vi "PH_ImageOperator.ProcCases.vi"(0 "i ref in":refnum<vi>, 1 "selector":string, 2 "data":T1, 3 "call cluster":T2={"Object"="", "Selector"="", "CallType"=enum."synchronous", "Async Object"="", "Async Selector"="", "Data Descriptor"="", "Data"=[], "Error #"=0, "Expire"=0}, 5 "error in":errorcluster) -> (14 "i ref out":refnum<vi>, 17 "answer cluster":T2={"Object"="", "Selector"="", "CallType"=enum."synchronous", "Async Object"="", "Async Selector"="", "Data Descriptor"="", "Data"=[], "Error #"=0, "Expire"=0}, 19 "error out":errorcluster)   [LabVIEW 2014, in "PH_ImageOperator.lvlib"]
doc: "This method is called by a process from within the default case in the event loop. The methods of a class that are linked to events will be called from THIS method. Add your code here."
uses:
  PH_ImageOperator.lvlib
  CSCore/CSSystem/CoreDefs/CoreDefs.call_type.ctl
  CSCore/BaseProcess/BaseProcess.descriptor string definition.ctl
  CSCore/CSSystem/CoreDefs/CoreDefs.rawDataType.ctl
  CSCore/CSSystem/CoreLib/CoreLib.byte array 2 short.vi
  CSCore/CSSystem/CoreLib/CoreLib.byte array 2 double.vi
  CSCore/CSSystem/CoreLib/CoreLib.string 2 byte array.vi
  CSCore/CSSystem/CoreLib/CoreLib.byte array 2 int.vi
  CSCore/CSSystem/CoreLib/CoreLib.lvlib
  CSCore/BaseProcess/BaseProcess.lvlib
  CSCore/CAEObj/CAEObj.lvlib
  PH_PSDBWriter/PH_PSDBWriter.lvlib
  PH_Common/PH_Common.lvlib
  PH_Img_BaseClass/PH_Img_BaseClass.lvlib
  PH_Cam_BaseClass/PH_Cam_BaseClass.lvlib
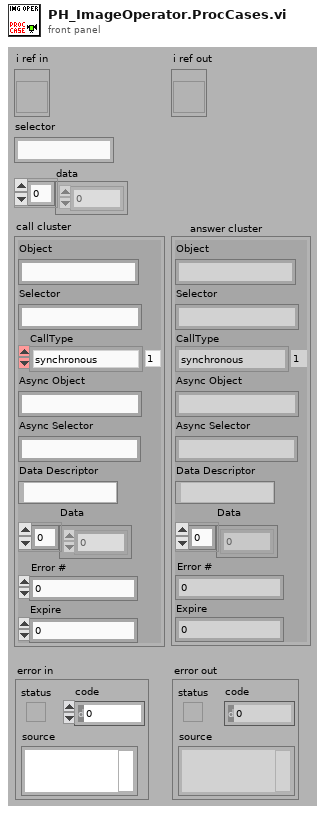
[diagram p1: front panel]
types:
  T1 = typedef "CoreDefs.rawDataType.ctl" = i8[]
  T2 = typedef "CoreDefs.call_type.ctl" = cluster{"Object":string, "Selector":string, "CallType":enum16{"simple", "synchronous", "asynchronous"}, "Async Object":string, "Async Selector":string, "Data Descriptor":T3, "Data":T1, "Error #":i32, "Expire":u32}
  T3 = typedef "BaseProcess.lvlib/BaseProcess.descriptor string definition.ctl" = string
  T4 = typedef "PH_Cam_BaseClass.lvlib/PH_Cam_BaseClass.Settings.ctl" = cluster{"Cam ID":string, "Gain":dbl, "Brightness":dbl, "Shutter":dbl, "Mode":i32}
  T5 = typedef "PH_ImageOperator.lvlib/PH_ImageOperator.i attribute.ctl" = cluster{"GUI Refs":cluster{"Delete":refnum<vi>, "Calibration status":refnum<vi>, "BI subtracted":refnum<vi>, "calc Energy":refnum<vi>, "Energy: expected value":refnum<vi>, "Energy: Tolerance":refnum<vi>, "Energy calculated":refnum<vi>, "Energy":refnum<vi>, "calc Beam Anal":refnum<vi>, "Maj Diam 1/esquare":refnum<vi>, "Min Diam 1/esquare":refnum<vi>, "Azi Angle":refnum<vi>, "Min/Maj Diam esquare":refnum<vi>, "Beam analysed":refnum<vi>, "CoG - x":refnum<vi>, "CoG - y":refnum<vi>, "BA: Method":refnum<vi>, "BA: Steps":refnum<vi>, "BA: Factor":refnum<vi>, "calc Traces":refnum<vi>, "Traces: Fit Gauss":refnum<vi>, "Traces calculated":refnum<vi>, "Maj FWHM":refnum<vi>, "Min FWHM":refnum<vi>, "Major Trace":refnum<vi>, "Minor Trace":refnum<vi>, "Maj Fit Order":refnum<vi>, "Min Fit Order":refnum<vi>, "Position calculated":refnum<vi>, "Position":refnum<vi>, "Type":refnum<vi>, "Center":refnum<vi>, "exp - X":refnum<vi>, "exp - Y":refnum<vi>, "Tolerance":refnum<vi>, "f":refnum<vi>, "M":refnum<vi>, "D":refnum<vi>, "q":refnum<vi>, "Dummy Method":refnum<vi>, "Dummy Type":refnum<vi>, "Global On":refnum<vi>, "Traces: No offset":refnum<vi>, "Maj 99%":refnum<vi>, "Min 99%":refnum<vi>, "GUI FF Image":refnum<vi>, "calc Fill Factor":refnum<vi>, "FF calculated":refnum<vi>, "Fill Factor: Filter?":refnum<vi>, "FF: Damage Threshold":refnum<vi>, "FF: Threshold":refnum<vi>, "FF: max allow. Energy":refnum<vi>, "FF: Fillfactor":refnum<vi>, "Calibration data":refnum<vi>}, "List of GUIs":string[], "Calibration":cluster{"Status":T6, "Calibration data":T7, "Calibration Data File":path}, "Final Image":cluster{"BI Subtraction Failure":bool}, "Energy":cluster{"on":bool, "expected value [mJ]":dbl, "Tolerance [%]":dbl, "State":T6, "Energy [mJ]":dbl, "Unit":string, "calculated @":timestamp}, "Beam Analysis":cluster{"on":bool, "Data":T8, "Method":bool, "Steps":i32, "Factor":i32, "ROI":cluster{"Left":i32, "Top":i32, "Right":i32, "Bottom":i32}, "analysed @":timestamp}, "Trace Analysis":cluster{"on":bool, "Fit on":bool, "Maj FWHM":dbl, "Min FWHM":dbl, "Maj Fit Order":i32, "Min Fit Order":i32, "No Offset":bool, "Maj 99%":dbl, "Min 99%":dbl, "Traces":cluster{"XScaleName":string, "Y Scale Minimum":sgl, "Y Scale Maximum":sgl, "X Scale Minimum":sgl, "X Scale Maximum":sgl, "Traces":cluster{"Index":sgl[], "Trace":dbl[]}[]}[], "analysed @":timestamp}, "Position Analysis":cluster{"on":bool, "exp - X":i32, "exp - Y":i32, "focal length [mm]":dbl, "Magnification":dbl, "Delta":dbl, "Theta":dbl, "Tolerance":dbl, "Type":bool, "analysed @":timestamp}, "Fill Factor":cluster{"on":bool, "Filter on?":bool, "Threshold":dbl, "Damage Threshold [J/cm²]":dbl, "Fillfactor":dbl, "Max. allowed Energy [J]":dbl, "calculated @":timestamp}, "Statistician Service ID":i32, "Images":cluster{"Background":T9, "OP":T9, "GUI":T9, "BA: ROI":T9, "Trace: Turn":T9, "FF: Main":T9, "FF: Help":T9, "PSDB: BG":T9, "PSDB: OP":T9, "PSDB: FF":T9}}
  T6 = typedef "PH_StatusHandler.lvlib/PH_StatusHandler.Status.ctl" = i16
  T7 = typedef "PH_ImageCalibrator.lvlib/PH_ImageCalibrator.Calibration Data.ctl" = cluster{"Date":string, "Time":string, "Cam Settings":cluster{"Cam ID":string, "Gain":dbl, "Brightness":dbl, "Shutter":dbl, "Cam Error":bool, "Mode":i32}, "Background Image":cluster{"Image":dbl[][], "Image Error":bool}, "Linear Calibration":cluster{"Calibration Factor":dbl, "not mm or mrad":bool}, "Energy Calibration":cluster{"Calibration Factor":dbl, "no mJ":bool}}
  T8 = typedef "PH_ImageOperator.lvlib/PH_ImageOperator.Beam Analysis Data.ctl" = cluster{"CoG-x":sgl, "CoG-y":sgl, "Maj Dim":dbl, "Min Dim":dbl, "Ellipticity":dbl, "Azimuth Angle [rad]":dbl, "Azi Angle rel to Maj?":bool}
  T9 = typedef "IMAQ Image.ctl" = refnum<image>
  T10 = typedef "PH_PSDBWriter.lvlib/PH_PSDBWriter.PHELIX-Subsystems.ctl" = i32
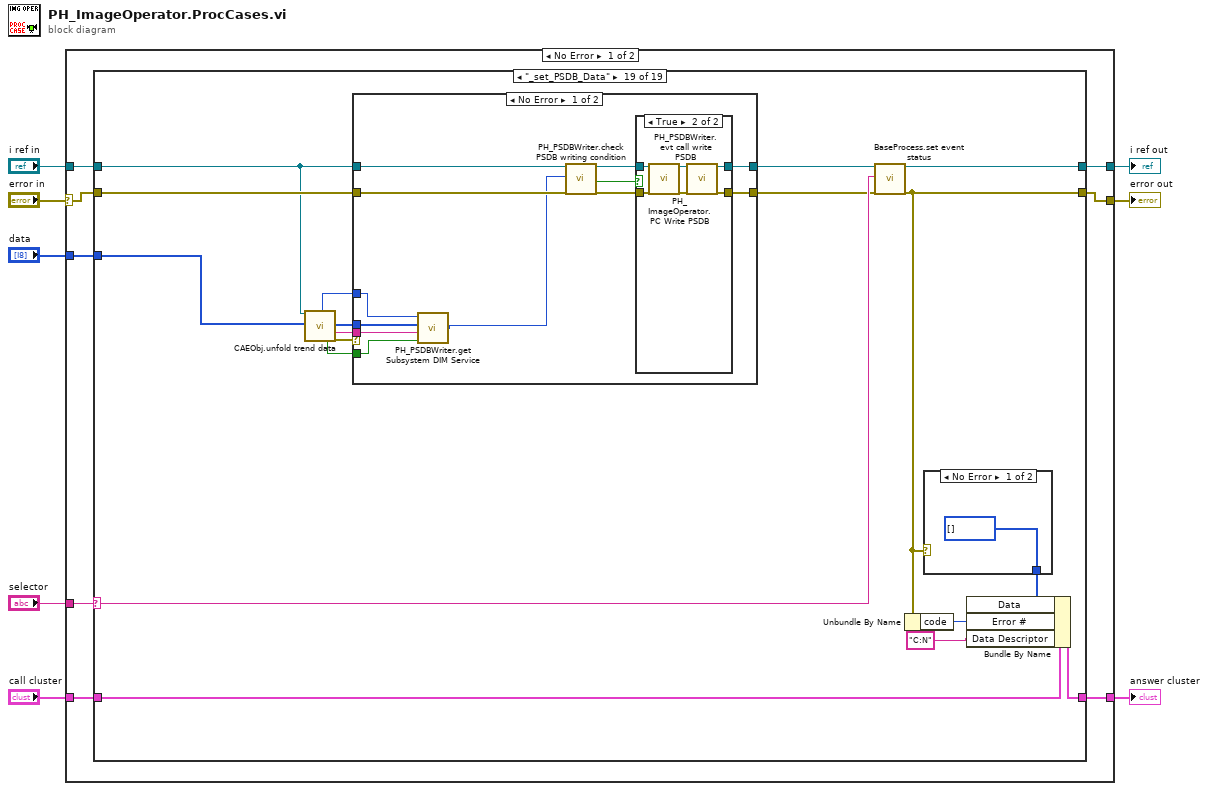
[diagram p0: block diagram]
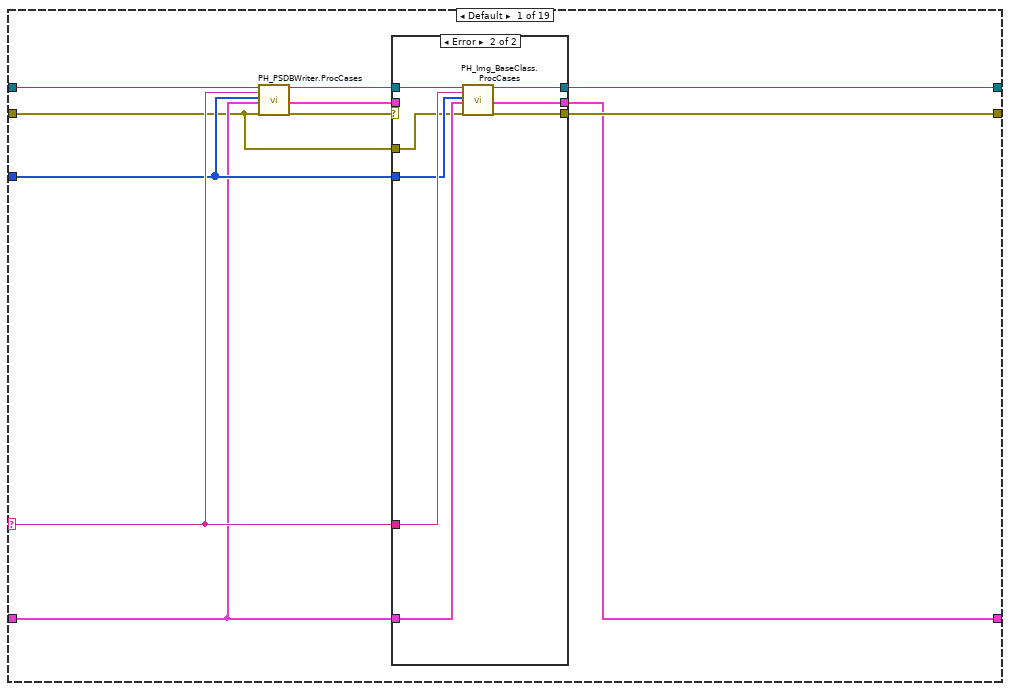
[diagram p2: hidden frame]
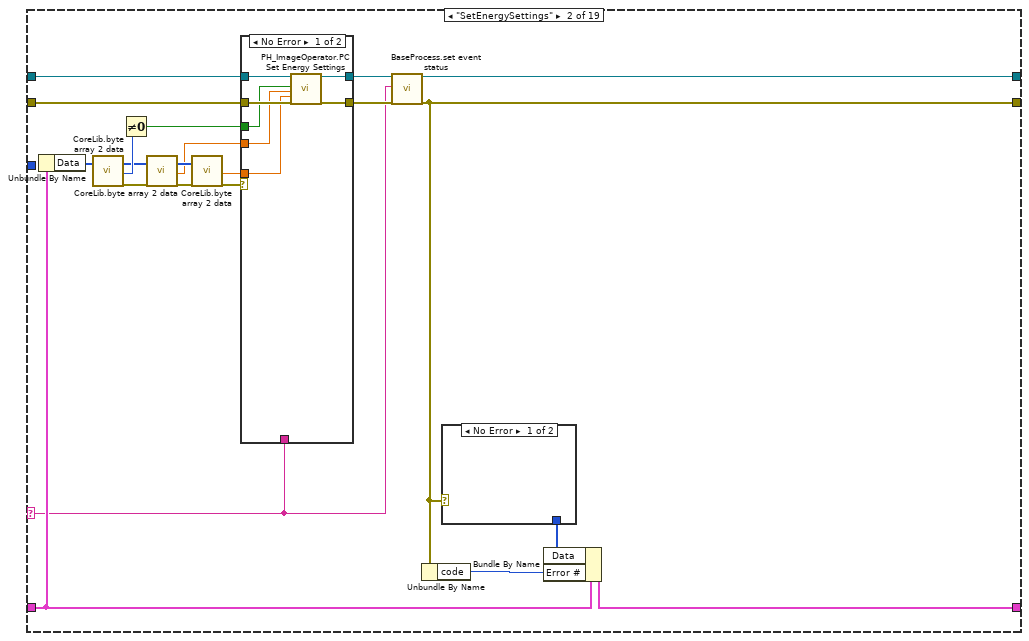
[diagram p4: hidden frame]
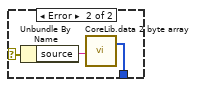
[diagram p5: hidden frame]
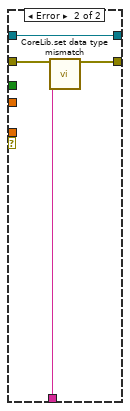
[diagram p6: hidden frame]
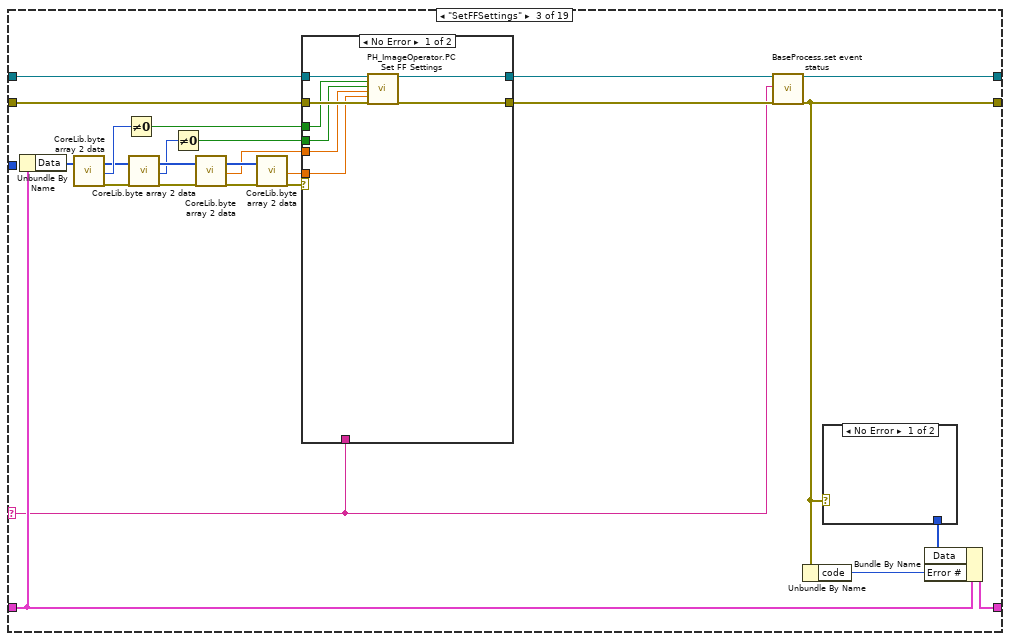
[diagram p7: hidden frame]
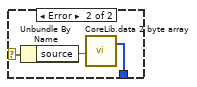
[diagram p8: hidden frame]
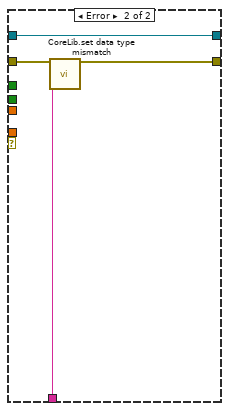
[diagram p9: hidden frame]
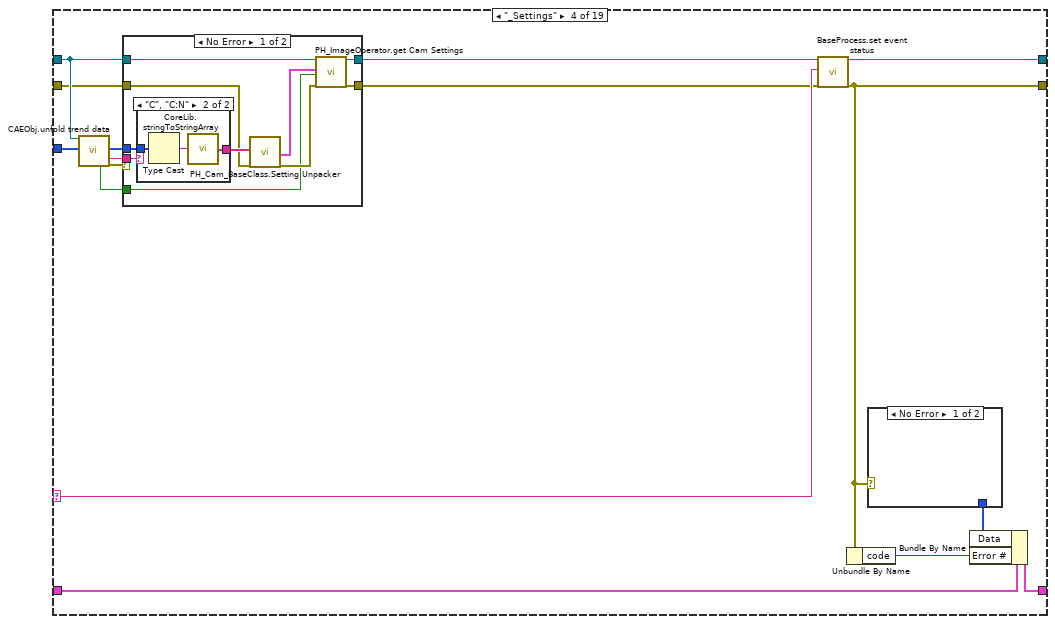
[diagram p10: hidden frame]
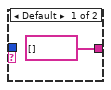
[diagram p11: hidden frame]
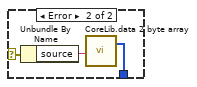
[diagram p13: hidden frame]
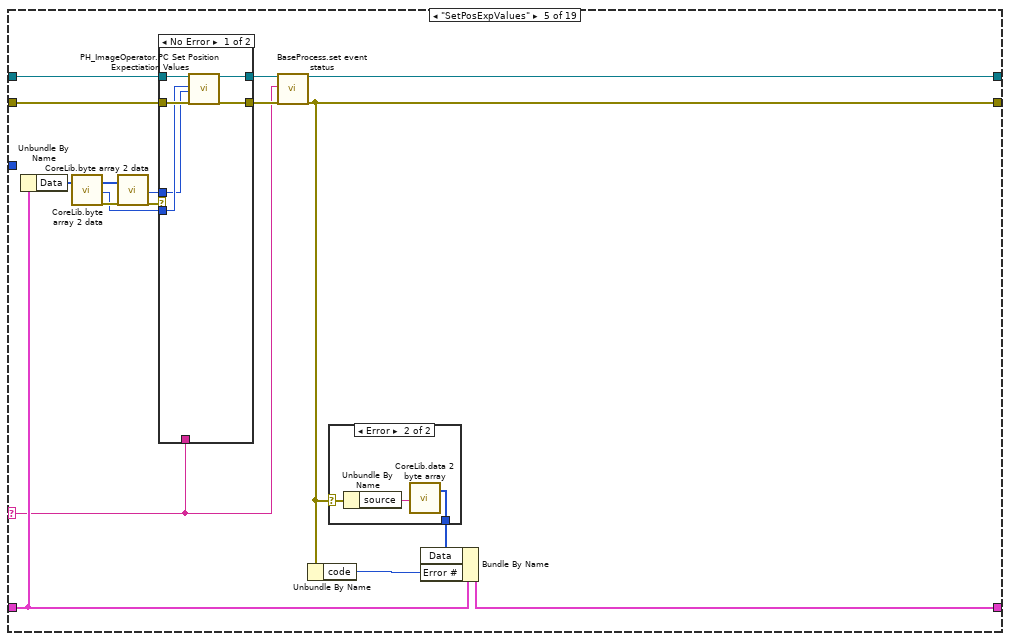
[diagram p14: hidden frame]
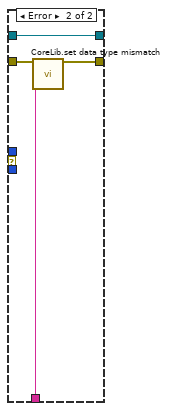
[diagram p16: hidden frame]
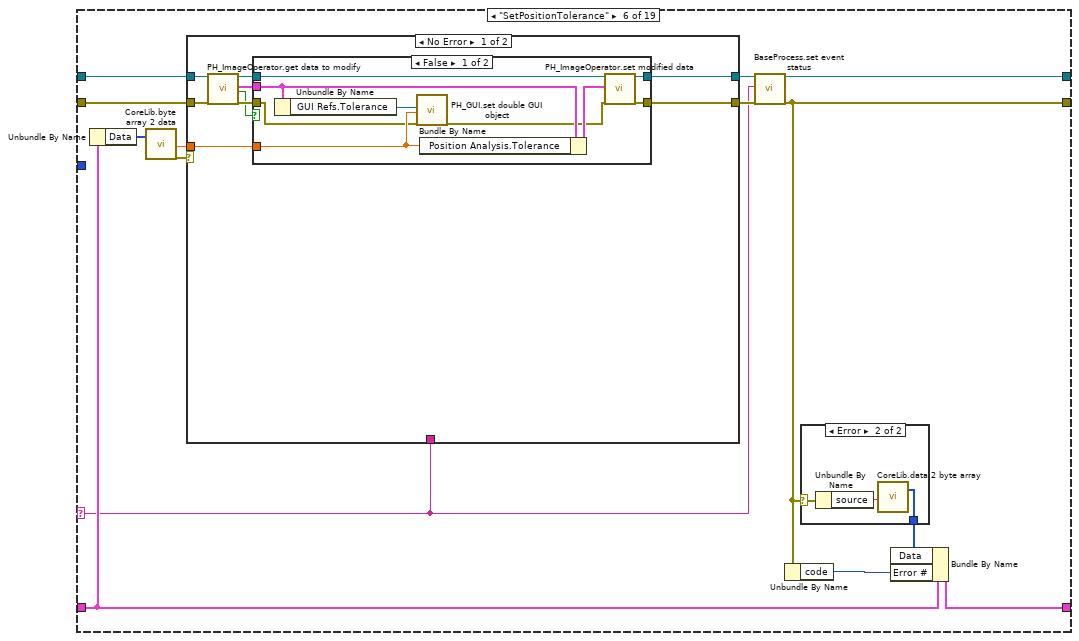
[diagram p17: hidden frame]
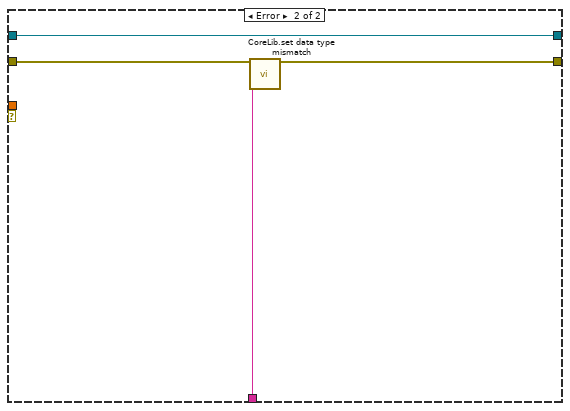
[diagram p20: hidden frame]
diagram:
  n1 = case shown="No Error" "error in" {
    selector: "error in" -> [w9 w619]
    tunnel: "selector" -> [w16 _]
    tunnel: [w15 w618] -> w7
    tunnel: "call cluster" -> [w14 w618]
    tunnel: "i ref in" -> [w13 w620]
    tunnel: [w12 w620] -> w5
    tunnel: [w11 w619] -> w4
    tunnel: "data" -> [w10 _]
    frame No Error {
      n2 = case shown="\"_set_PSDB_Data\"" w16 {
        selector: w16 -> [w22 w51 w90 w125 w157 w184 w225 w266 w314 w343 w370 w397 w424 w464 w485 w512 w539 w566 w586]
        tunnel: w10 -> [w21 _ _ w114 _ _ _ _ _ _ _ _ _ _ _ _ _ _ w574]
        tunnel: w13 -> [w27 w59 w98 w118 w165 w192 w233 w274 w322 w351 w378 w405 w432 w462 w493 w520 w547 w564 w577]
        tunnel: [w24 w50 w89 w124 w156 w183 w224 w265 w313 w342 w369 w396 w423 w463 w484 w511 w538 w565 w587] -> w12
        tunnel: w14 -> [w20 w56 w95 w128 w162 w189 w230 w271 w319 w348 w375 w402 w429 w469 w490 w517 w544 w569 w590]
        tunnel: [w18 w55 w94 w127 w161 w188 w229 w270 w318 w347 w374 w401 w428 w468 w489 w516 w543 w568 w589] -> w15
        tunnel: w9 -> [w17 w58 w97 w116 w164 w191 w232 w273 w321 w350 w377 w404 w431 w460 w492 w519 w546 w563 w578]
        tunnel: [w26 w52 w91 w126 w158 w185 w226 w267 w315 w344 w371 w398 w425 w465 w486 w513 w540 w567 w588] -> w11
        frame Default {
          n3 = call "PH_PSDBWriter.ProcCases.vi"("i ref in"=w27, "selector"=w22, "Data"=w21, "call cluster"=w20, "error in"=w17) -> ("i ref out"=w25:refnum<vi>, "answer cluster"=w19:T2, "error out"=w23:errorcluster)  [unwired: 12 in]
          n4 = case shown="Error" w23 {
            selector: w23 -> [w29 _]
            tunnel: [w29 w38] -> w26
            tunnel: w25 -> [w30 w37]
            tunnel: [w30 w36] -> w24
            tunnel: w22 -> [_ w35]
            tunnel: w21 -> [_ w34]
            tunnel: w20 -> [_ w33]
            tunnel: [w28 w32] -> w18
            tunnel: w19 -> [w28 _]
            tunnel: w17 -> [_ w31]
            frame No Error {
            }
            frame Error {
              n5 = call "PH_Img_BaseClass.ProcCases.vi"("i ref in"=w37, "selector"=w35, "Data"=w34, "call cluster"=w33, "error in (no error)"=w31) -> ("i ref out"=w36:refnum<vi>, "answer cluster"=w32:T2, "error out"=w38:errorcluster)  [unwired: 12 in]
            }
          }
        }
        frame "SetEnergySettings" {
          n6 = Unbundle By Name(w56) -> ("Data"=w39:T1)
          n7 = call-poly "CoreLib.byte array 2 data.vi"("byteArray"=w39) -> ("byteArray out"=w45:T1, "i16"=w48:i16, "error out"=w44:errorcluster)  [unwired: 16 in]
          n8 = Not Equal To 0?(x=w48) -> (x != 0?=w41:bool)
          n9 = call-poly "CoreLib.byte array 2 data.vi"("byteArray"=w45, "error in (no error)"=w44) -> ("byteArray out"=w47:T1, "d64"=w43:dbl, "error out"=w46:errorcluster)  [unwired: 15 in]
          n10 = call-poly "CoreLib.byte array 2 data.vi"("byteArray"=w47, "error in (no error)"=w46) -> ("d64"=w42:dbl, "error out"=w40:errorcluster)  [unwired: 15 in, 1 out]
          n11 = case shown="No Error" w40 {
            tunnel: [w68 w73] -> w54
            tunnel: w59 -> [w69 w73]
            tunnel: w58 -> [w67 w72]
            tunnel: [w66 w71] -> w53
            tunnel: w43 -> [w64 _]
            tunnel: w51 -> [_ w70]
            tunnel: w41 -> [w65 _]
            tunnel: w42 -> [w63 _]
            frame No Error {
              n12 = call "PH_ImageOperator.PC Set Energy Settings.vi"("i ref in"=w69, "Calc Energy"=w65, "Expected Value [mJ]"=w64, "Tolerance [%]"=w63, "error in (no error)"=w67) -> ("i ref out"=w68:refnum<vi>, "error out"=w66:errorcluster)  [unwired: 13 in]
            }
            frame Error {
              n13 = call "CoreLib.set data type mismatch.vi"("error in (no error)"=w72, "error source"=w70) -> ("error out"=w71:errorcluster)  [unwired: 17 in]
            }
          }
          n14 = call "BaseProcess.set event status.vi"("i ref in"=w54, "EventStatus"=w51, "error in (no error)"=w53) -> ("i ref out"=w50:refnum<vi>, "error out"=w52:errorcluster)  [unwired: 14 in, 1 out]
          n15 = Unbundle By Name(w52) -> ("code"=w57:i32)
          n16 = case shown="No Error" w52 {
            selector: w52 -> [_ w62]
            tunnel: [_ w60] -> w49
            frame No Error {
            }
            frame Error {
              n17 = Unbundle By Name(w62) -> ("source"=w61:string)
              n18 = call-poly "CoreLib.data 2 byte array.vi"("string"=w61) -> ("byteArray out"=w60:T1)  [unwired: 18 in]
            }
          }
          n19 = Bundle By Name(cluster=w56, "Data"=w49, "Error #"=w57) -> (w55:T2)
        }
        frame "SetFFSettings" {
          n20 = Unbundle By Name(w95) -> ("Data"=w80:T1)
          n21 = call-poly "CoreLib.byte array 2 data.vi"("byteArray"=w80) -> ("byteArray out"=w77:T1, "i16"=w87:i16, "error out"=w79:errorcluster)  [unwired: 16 in]
          n22 = Not Equal To 0?(x=w87) -> (x != 0?=w82:bool)
          n23 = call-poly "CoreLib.byte array 2 data.vi"("byteArray"=w77, "error in (no error)"=w79) -> ("byteArray out"=w76:T1, "i16"=w75:i16, "error out"=w78:errorcluster)  [unwired: 15 in]
          n24 = Not Equal To 0?(x=w75) -> (x != 0?=w74:bool)
          n25 = call-poly "CoreLib.byte array 2 data.vi"("byteArray"=w76, "error in (no error)"=w78) -> ("byteArray out"=w86:T1, "d64"=w84:dbl, "error out"=w85:errorcluster)  [unwired: 15 in]
          n26 = call-poly "CoreLib.byte array 2 data.vi"("byteArray"=w86, "error in (no error)"=w85) -> ("d64"=w83:dbl, "error out"=w81:errorcluster)  [unwired: 15 in, 1 out]
          n27 = case shown="No Error" w81 {
            tunnel: [w108 w113] -> w93
            tunnel: w98 -> [w109 w113]
            tunnel: w97 -> [w107 w112]
            tunnel: [w106 w111] -> w92
            tunnel: w84 -> [w105 _]
            tunnel: w90 -> [_ w110]
            tunnel: w82 -> [w103 _]
            tunnel: w83 -> [w104 _]
            tunnel: w74 -> [w102 _]
            frame No Error {
              n28 = call "PH_ImageOperator.PC Set FF Settings.vi"("i ref in"=w109, "Calc Fill Factor"=w103, "Filter"=w102, "Threshold"=w105, "Damage Threshold [J/cm²]"=w104, "error in (no error)"=w107) -> ("i ref out"=w108:refnum<vi>, "error out"=w106:errorcluster)  [unwired: 12 in]
            }
            frame Error {
              n29 = call "CoreLib.set data type mismatch.vi"("error in (no error)"=w112, "error source"=w110) -> ("error out"=w111:errorcluster)  [unwired: 17 in]
            }
          }
          n30 = call "BaseProcess.set event status.vi"("i ref in"=w93, "EventStatus"=w90, "error in (no error)"=w92) -> ("i ref out"=w89:refnum<vi>, "error out"=w91:errorcluster)  [unwired: 14 in, 1 out]
          n31 = Unbundle By Name(w91) -> ("code"=w96:i32)
          n32 = case shown="No Error" w91 {
            selector: w91 -> [_ w101]
            tunnel: [_ w99] -> w88
            frame No Error {
            }
            frame Error {
              n33 = Unbundle By Name(w101) -> ("source"=w100:string)
              n34 = call-poly "CoreLib.data 2 byte array.vi"("string"=w100) -> ("byteArray out"=w99:T1)  [unwired: 18 in]
            }
          }
          n35 = Bundle By Name(cluster=w95, "Data"=w88, "Error #"=w96) -> (w94:T2)
        }
        frame "_Settings" {
          n36 = call "CAEObj.unfold trend data.vi"("i ref in"=w118, "raw trend data"=w114) -> ("no link"=w119:bool, "data"=w120:i8[], "typeDescriptor"=w121:string, "error out"=w122:errorcluster)  [unwired: 9 in, 5 out]
          n37 = case shown="No Error" w122 {
            tunnel: w118 -> [w134 w145]
            tunnel: [w132 w145] -> w117
            tunnel: w116 -> [w136 w144]
            tunnel: [w133 w144] -> w115
            tunnel: w121 -> [w139 _]
            tunnel: w120 -> [w138 _]
            tunnel: w119 -> [w130 _]
            frame No Error {
              n38 = case shown="\"C\", \"C:N\"" w139 {
                tunnel: w138 -> [_ w143]
                tunnel: [string[] [] ("Array") w141] -> w137
                frame Default {
                }
                frame "C", "C:N" {
                  n39 = Type Cast(x=w143) -> (*(type *) &x=w142:string)  [unwired: 1 in]
                  n40 = call "CoreLib.stringToStringArray.vi"("String"=w142) -> ("Array"=w141:string[])
                }
              }
              n41 = call "PH_Cam_BaseClass.Setting Unpacker.vi"("Cam Settings Array"=w137, "error in (no error)"=w136) -> ("Cam Settings"=w131:T4, "error out"=w135:errorcluster)  [unwired: 15 in, 1 out]
              n42 = call "PH_ImageOperator.get Cam Settings.vi"("i ref in"=w134, "Cam Settings"=w131, "Cam Info Failure"=w130, "error in (no error)"=w135) -> ("i ref out"=w132:refnum<vi>, "error out"=w133:errorcluster)  [unwired: 14 in]
            }
            frame Error {
            }
          }
          n43 = call "BaseProcess.set event status.vi"("i ref in"=w117, "EventStatus"=w125, "error in (no error)"=w115) -> ("i ref out"=w124:refnum<vi>, "error out"=w126:errorcluster)  [unwired: 14 in, 1 out]
          n44 = Unbundle By Name(w126) -> ("code"=w129:i32)
          n45 = case shown="No Error" w126 {
            selector: w126 -> [_ w148]
            tunnel: [_ w146] -> w123
            frame No Error {
            }
            frame Error {
              n46 = Unbundle By Name(w148) -> ("source"=w147:string)
              n47 = call-poly "CoreLib.data 2 byte array.vi"("string"=w147) -> ("byteArray out"=w146:T1)  [unwired: 18 in]
            }
          }
          n48 = Bundle By Name(cluster=w128, "Data"=w123, "Error #"=w129) -> (w127:T2)
        }
        frame "SetPosExpValues" {
          n49 = Unbundle By Name(w162) -> ("Data"=w150:T1)
          n50 = call-poly "CoreLib.byte array 2 data.vi"("byteArray"=w150) -> ("byteArray out"=w155:T1, "i32"=w153:i32, "error out"=w154:errorcluster)  [unwired: 16 in]
          n51 = call-poly "CoreLib.byte array 2 data.vi"("byteArray"=w155, "error in (no error)"=w154) -> ("i32"=w152:i32, "error out"=w151:errorcluster)  [unwired: 15 in, 1 out]
          n52 = case shown="No Error" w151 {
            tunnel: [w173 w178] -> w160
            tunnel: w165 -> [w174 w178]
            tunnel: w164 -> [w172 w177]
            tunnel: [w171 w176] -> w159
            tunnel: w153 -> [w170 _]
            tunnel: w157 -> [_ w175]
            tunnel: w152 -> [w169 _]
            frame No Error {
              n53 = call "PH_ImageOperator.PC Set Position Expectiation Values.vi"("i ref in"=w174, "expected X"=w170, "expected Y"=w169, "error in (no error)"=w172) -> ("i ref out"=w173:refnum<vi>, "error out"=w171:errorcluster)  [unwired: 14 in]
            }
            frame Error {
              n54 = call "CoreLib.set data type mismatch.vi"("error in (no error)"=w177, "error source"=w175) -> ("error out"=w176:errorcluster)  [unwired: 17 in]
            }
          }
          n55 = call "BaseProcess.set event status.vi"("i ref in"=w160, "EventStatus"=w157, "error in (no error)"=w159) -> ("i ref out"=w156:refnum<vi>, "error out"=w158:errorcluster)  [unwired: 14 in, 1 out]
          n56 = Unbundle By Name(w158) -> ("code"=w163:i32)
          n57 = case shown="Error" w158 {
            selector: w158 -> [_ w168]
            tunnel: [_ w166] -> w149
            frame No Error {
            }
            frame Error {
              n58 = Unbundle By Name(w168) -> ("source"=w167:string)
              n59 = call-poly "CoreLib.data 2 byte array.vi"("string"=w167) -> ("byteArray out"=w166:T1)  [unwired: 18 in]
            }
          }
          n60 = Bundle By Name(cluster=w162, "Data"=w149, "Error #"=w163) -> (w161:T2)
        }
        frame "SetPositionTolerance" {
          n61 = Unbundle By Name(w189) -> ("Data"=w180:T1)
          n62 = call-poly "CoreLib.byte array 2 data.vi"("byteArray"=w180) -> ("d64"=w182:dbl, "error out"=w181:errorcluster)  [unwired: 16 in, 1 out]
          n63 = case shown="No Error" w181 {
            tunnel: [w200 w219] -> w187
            tunnel: w192 -> [w204 w219]
            tunnel: w191 -> [w203 w218]
            tunnel: [w199 w217] -> w186
            tunnel: w182 -> [w197 _]
            tunnel: w184 -> [_ w216]
            frame No Error {
              n64 = call "PH_ImageOperator.get data to modify.vi"("i ref in"=w204, "error in (no error)"=w203) -> ("i ref out"=w201:refnum<vi>, "i attribute"=w198:T5, "timed out"=w196:bool, "error out"=w202:errorcluster)  [unwired: 14 in]
              n65 = case shown="False" w196 {
                tunnel: w202 -> [w206 w214]
                tunnel: w201 -> [w213 w215]
                tunnel: [w212 w215] -> w200
                tunnel: [w211 w214] -> w199
                tunnel: w198 -> [w209 _]
                tunnel: w197 -> [w207 _]
                frame False {
                  n66 = Unbundle By Name(w209) -> ("GUI Refs.Tolerance"=w208:refnum<vi>)
                  n67 = call "PH_GUI.set double GUI object.vi"("GUI object Ref"=w208, "value"=w207, "error in (no error)"=w206) -> ("error out"=w205:errorcluster)  [unwired: 16 in]
                  n68 = Bundle By Name(cluster=w209, "Position Analysis.Tolerance"=w207) -> (w210:T5)
                  n69 = call "PH_ImageOperator.set modified data.vi"("i ref in"=w213, "i attribute"=w210, "error in (no error)"=w205) -> ("i ref out"=w212:refnum<vi>, "error out"=w211:errorcluster)  [unwired: 15 in]
                }
                frame True {
                }
              }
            }
            frame Error {
              n70 = call "CoreLib.set data type mismatch.vi"("error in (no error)"=w218, "error source"=w216) -> ("error out"=w217:errorcluster)  [unwired: 17 in]
            }
          }
          n71 = call "BaseProcess.set event status.vi"("i ref in"=w187, "EventStatus"=w184, "error in (no error)"=w186) -> ("i ref out"=w183:refnum<vi>, "error out"=w185:errorcluster)  [unwired: 14 in, 1 out]
          n72 = Unbundle By Name(w185) -> ("code"=w190:i32)
          n73 = case shown="Error" w185 {
            selector: w185 -> [_ w195]
            tunnel: [_ w193] -> w179
            frame No Error {
            }
            frame Error {
              n74 = Unbundle By Name(w195) -> ("source"=w194:string)
              n75 = call-poly "CoreLib.data 2 byte array.vi"("string"=w194) -> ("byteArray out"=w193:T1)  [unwired: 18 in]
            }
          }
          n76 = Bundle By Name(cluster=w189, "Data"=w179, "Error #"=w190) -> (w188:T2)
        }
        frame "SetFocalLength" {
          n77 = Unbundle By Name(w230) -> ("Data"=w223:T1)
          n78 = call-poly "CoreLib.byte array 2 data.vi"("byteArray"=w223) -> ("d64"=w222:dbl, "error out"=w221:errorcluster)  [unwired: 16 in, 1 out]
          n79 = case shown="No Error" w221 {
            tunnel: [w241 w260] -> w228
            tunnel: w233 -> [w245 w260]
            tunnel: w232 -> [w244 w259]
            tunnel: [w240 w258] -> w227
            tunnel: w222 -> [w238 _]
            tunnel: w225 -> [_ w257]
            frame No Error {
              n80 = call "PH_ImageOperator.get data to modify.vi"("i ref in"=w245, "error in (no error)"=w244) -> ("i ref out"=w242:refnum<vi>, "i attribute"=w239:T5, "timed out"=w237:bool, "error out"=w243:errorcluster)  [unwired: 14 in]
              n81 = case shown="False" w237 {
                tunnel: w243 -> [w247 w255]
                tunnel: w242 -> [w254 w256]
                tunnel: [w253 w256] -> w241
                tunnel: [w252 w255] -> w240
                tunnel: w239 -> [w250 _]
                tunnel: w238 -> [w248 _]
                frame False {
                  n82 = Unbundle By Name(w250) -> ("GUI Refs.f"=w249:refnum<vi>)
                  n83 = Bundle By Name(cluster=w250, "Position Analysis.focal length [mm]"=w248) -> (w251:T5)
                  n84 = call "PH_GUI.set double GUI object.vi"("GUI object Ref"=w249, "value"=w248, "error in (no error)"=w247) -> ("error out"=w246:errorcluster)  [unwired: 16 in]
                  n85 = call "PH_ImageOperator.set modified data.vi"("i ref in"=w254, "i attribute"=w251, "error in (no error)"=w246) -> ("i ref out"=w253:refnum<vi>, "error out"=w252:errorcluster)  [unwired: 15 in]
                }
                frame True {
                }
              }
            }
            frame Error {
              n86 = call "CoreLib.set data type mismatch.vi"("error in (no error)"=w259, "error source"=w257) -> ("error out"=w258:errorcluster)  [unwired: 17 in]
            }
          }
          n87 = call "BaseProcess.set event status.vi"("i ref in"=w228, "EventStatus"=w225, "error in (no error)"=w227) -> ("i ref out"=w224:refnum<vi>, "error out"=w226:errorcluster)  [unwired: 14 in, 1 out]
          n88 = Unbundle By Name(w226) -> ("code"=w231:i32)
          n89 = case shown="Error" w226 {
            selector: w226 -> [_ w236]
            tunnel: [_ w234] -> w220
            frame No Error {
            }
            frame Error {
              n90 = Unbundle By Name(w236) -> ("source"=w235:string)
              n91 = call-poly "CoreLib.data 2 byte array.vi"("string"=w235) -> ("byteArray out"=w234:T1)  [unwired: 18 in]
            }
          }
          n92 = Bundle By Name(cluster=w230, "Data"=w220, "Error #"=w231) -> (w229:T2)
        }
        frame "SetMagnification" {
          n93 = Unbundle By Name(w271) -> ("Data"=w264:T1)
          n94 = call-poly "CoreLib.byte array 2 data.vi"("byteArray"=w264) -> ("d64"=w263:dbl, "error out"=w262:errorcluster)  [unwired: 16 in, 1 out]
          n95 = case shown="No Error" w262 {
            tunnel: [w282 w301] -> w269
            tunnel: w274 -> [w286 w301]
            tunnel: w273 -> [w285 w300]
            tunnel: [w281 w299] -> w268
            tunnel: w263 -> [w279 _]
            tunnel: w266 -> [_ w298]
            frame No Error {
              n96 = call "PH_ImageOperator.get data to modify.vi"("i ref in"=w286, "error in (no error)"=w285) -> ("i ref out"=w283:refnum<vi>, "i attribute"=w280:T5, "timed out"=w278:bool, "error out"=w284:errorcluster)  [unwired: 14 in]
              n97 = case shown="False" w278 {
                tunnel: w284 -> [w290 w296]
                tunnel: w283 -> [w295 w297]
                tunnel: [w294 w297] -> w282
                tunnel: [w293 w296] -> w281
                tunnel: w280 -> [w291 _]
                tunnel: w279 -> [w287 _]
                frame False {
                  n98 = Unbundle By Name(w291) -> ("GUI Refs.M"=w288:refnum<vi>)
                  n99 = call "PH_GUI.set double GUI object.vi"("GUI object Ref"=w288, "value"=w287, "error in (no error)"=w290) -> ("error out"=w289:errorcluster)  [unwired: 16 in]
                  n100 = Bundle By Name(cluster=w291, "Position Analysis.Magnification"=w287) -> (w292:T5)
                  n101 = call "PH_ImageOperator.set modified data.vi"("i ref in"=w295, "i attribute"=w292, "error in (no error)"=w289) -> ("i ref out"=w294:refnum<vi>, "error out"=w293:errorcluster)  [unwired: 15 in]
                }
                frame True {
                }
              }
            }
            frame Error {
              n102 = call "CoreLib.set data type mismatch.vi"("error in (no error)"=w300, "error source"=w298) -> ("error out"=w299:errorcluster)  [unwired: 17 in]
            }
          }
          n103 = call "BaseProcess.set event status.vi"("i ref in"=w269, "EventStatus"=w266, "error in (no error)"=w268) -> ("i ref out"=w265:refnum<vi>, "error out"=w267:errorcluster)  [unwired: 14 in, 1 out]
          n104 = Unbundle By Name(w267) -> ("code"=w272:i32)
          n105 = case shown="Error" w267 {
            selector: w267 -> [_ w277]
            tunnel: [_ w275] -> w261
            frame No Error {
              (unwired) ""
            }
            frame Error {
              n106 = Unbundle By Name(w277) -> ("source"=w276:string)
              n107 = call-poly "CoreLib.data 2 byte array.vi"("string"=w276) -> ("byteArray out"=w275:T1)  [unwired: 18 in]
            }
          }
          n108 = Bundle By Name(cluster=w271, "Data"=w261, "Error #"=w272) -> (w270:T2)
        }
        frame "SetAnalysisMethod" {
          n109 = Unbundle By Name(w319) -> ("Data"=w306:T1)
          n110 = call-poly "CoreLib.byte array 2 data.vi"("byteArray"=w306) -> ("byteArray out"=w308:T1, "i16"=w311:i16, "error out"=w307:errorcluster)  [unwired: 16 in]
          n111 = call-poly "CoreLib.byte array 2 data.vi"("byteArray"=w308, "error in (no error)"=w307) -> ("byteArray out"=w310:T1, "i32"=w304:i32, "error out"=w309:errorcluster)  [unwired: 15 in]
          n112 = Not Equal To 0?(x=w311) -> (x != 0?=w305:bool)
          n113 = call-poly "CoreLib.byte array 2 data.vi"("byteArray"=w310, "error in (no error)"=w309) -> ("i32"=w303:i32, "error out"=w302:errorcluster)  [unwired: 15 in, 1 out]
          n114 = case shown="No Error" w302 {
            tunnel: [w331 w336] -> w317
            tunnel: w322 -> [w332 w336]
            tunnel: w321 -> [w330 w335]
            tunnel: [w329 w334] -> w316
            tunnel: w304 -> [w327 _]
            tunnel: w314 -> [_ w333]
            tunnel: w305 -> [w328 _]
            tunnel: w303 -> [w326 _]
            frame No Error {
              n115 = call "PH_ImageOperator.PC Set Analysis Method.vi"("i ref in"=w332, "Over All / Iterative"=w328, "Steps (3)"=w327, "Factor of ROI (3)"=w326, "error in (no error)"=w330) -> ("i ref out"=w331:refnum<vi>, "error out"=w329:errorcluster)  [unwired: 13 in]
            }
            frame Error {
              n116 = call "CoreLib.set data type mismatch.vi"("error in (no error)"=w335, "error source"=w333) -> ("error out"=w334:errorcluster)  [unwired: 17 in]
            }
          }
          n117 = call "BaseProcess.set event status.vi"("i ref in"=w317, "EventStatus"=w314, "error in (no error)"=w316) -> ("i ref out"=w313:refnum<vi>, "error out"=w315:errorcluster)  [unwired: 14 in, 1 out]
          n118 = Unbundle By Name(w315) -> ("code"=w320:i32)
          n119 = case shown="Error" w315 {
            selector: w315 -> [_ w325]
            tunnel: [_ w323] -> w312
            frame No Error {
            }
            frame Error {
              n120 = Unbundle By Name(w325) -> ("source"=w324:string)
              n121 = call-poly "CoreLib.data 2 byte array.vi"("string"=w324) -> ("byteArray out"=w323:T1)  [unwired: 18 in]
            }
          }
          n122 = Bundle By Name(cluster=w319, "Data"=w312, "Error #"=w320) -> (w318:T2)
        }
        frame "SetBeamAnalysis" {
          n123 = Unbundle By Name(w348) -> ("Data"=w340:T1)
          n124 = call-poly "CoreLib.byte array 2 data.vi"("byteArray"=w340) -> ("i16"=w341:i16, "error out"=w338:errorcluster)  [unwired: 16 in, 1 out]
          n125 = Not Equal To 0?(x=w341) -> (x != 0?=w339:bool)
          n126 = case shown="No Error" w338 {
            tunnel: [w357 w363] -> w346
            tunnel: w351 -> [w359 w363]
            tunnel: w350 -> [w358 w362]
            tunnel: [w356 w361] -> w345
            tunnel: w343 -> [_ w360]
            tunnel: w339 -> [w355 _]
            frame No Error {
              n127 = call "PH_ImageOperator.PC Set Beam Analysis.vi"("i ref in"=w359, "On / Off"=w355, "error in"=w358) -> ("i ref out"=w357:refnum<vi>, "error out"=w356:errorcluster)  [unwired: 15 in]
            }
            frame Error {
              n128 = call "CoreLib.set data type mismatch.vi"("error in (no error)"=w362, "error source"=w360) -> ("error out"=w361:errorcluster)  [unwired: 17 in]
            }
          }
          n129 = call "BaseProcess.set event status.vi"("i ref in"=w346, "EventStatus"=w343, "error in (no error)"=w345) -> ("i ref out"=w342:refnum<vi>, "error out"=w344:errorcluster)  [unwired: 14 in, 1 out]
          n130 = Unbundle By Name(w344) -> ("code"=w349:i32)
          n131 = case shown="Error" w344 {
            selector: w344 -> [_ w354]
            tunnel: [_ w352] -> w337
            frame No Error {
            }
            frame Error {
              n132 = Unbundle By Name(w354) -> ("source"=w353:string)
              n133 = call-poly "CoreLib.data 2 byte array.vi"("string"=w353) -> ("byteArray out"=w352:T1)  [unwired: 18 in]
            }
          }
          n134 = Bundle By Name(cluster=w348, "Data"=w337, "Error #"=w349) -> (w347:T2)
        }
        frame "GlobalOn" {
          n135 = Unbundle By Name(w375) -> ("Data"=w365:T1)
          n136 = call-poly "CoreLib.byte array 2 data.vi"("byteArray"=w365) -> ("i16"=w368:i16, "error out"=w366:errorcluster)  [unwired: 16 in, 1 out]
          n137 = Not Equal To 0?(x=w368) -> (x != 0?=w367:bool)
          n138 = case shown="No Error" w366 {
            tunnel: [w386 w390] -> w373
            tunnel: w378 -> [w384 w390]
            tunnel: w377 -> [w383 w389]
            tunnel: [w385 w388] -> w372
            tunnel: w370 -> [_ w387]
            tunnel: w367 -> [w382 _]
            frame No Error {
              n139 = call "PH_ImageOperator.PC set Global On.vi"("i ref in"=w384, "Global On"=w382, "error in (no error)"=w383) -> ("i ref out"=w386:refnum<vi>, "error out"=w385:errorcluster)  [unwired: 15 in]
            }
            frame Error {
              n140 = call "CoreLib.set data type mismatch.vi"("error in (no error)"=w389, "error source"=w387) -> ("error out"=w388:errorcluster)  [unwired: 17 in]
            }
          }
          n141 = call "BaseProcess.set event status.vi"("i ref in"=w373, "EventStatus"=w370, "error in (no error)"=w372) -> ("i ref out"=w369:refnum<vi>, "error out"=w371:errorcluster)  [unwired: 14 in, 1 out]
          n142 = Unbundle By Name(w371) -> ("code"=w376:i32)
          n143 = case shown="Error" w371 {
            selector: w371 -> [_ w381]
            tunnel: [_ w379] -> w364
            frame No Error {
            }
            frame Error {
              n144 = Unbundle By Name(w381) -> ("source"=w380:string)
              n145 = call-poly "CoreLib.data 2 byte array.vi"("string"=w380) -> ("byteArray out"=w379:T1)  [unwired: 18 in]
            }
          }
          n146 = Bundle By Name(cluster=w375, "Data"=w364, "Error #"=w376) -> (w374:T2)
        }
        frame "PositionOn" {
          n147 = Unbundle By Name(w402) -> ("Data"=w394:T1)
          n148 = call-poly "CoreLib.byte array 2 data.vi"("byteArray"=w394) -> ("i16"=w395:i16, "error out"=w392:errorcluster)  [unwired: 16 in, 1 out]
          n149 = Not Equal To 0?(x=w395) -> (x != 0?=w393:bool)
          n150 = case shown="No Error" w392 {
            tunnel: [w410 w417] -> w400
            tunnel: w405 -> [w413 w417]
            tunnel: w404 -> [w412 w416]
            tunnel: [w411 w415] -> w399
            tunnel: w397 -> [_ w414]
            tunnel: w393 -> [w409 _]
            frame No Error {
              n151 = call "PH_ImageOperator.PC set Position On.vi"("i ref in"=w413, "Position on"=w409, "error in (no error)"=w412) -> ("i ref out"=w410:refnum<vi>, "error out"=w411:errorcluster)  [unwired: 15 in]
            }
            frame Error {
              n152 = call "CoreLib.set data type mismatch.vi"("error in (no error)"=w416, "error source"=w414) -> ("error out"=w415:errorcluster)  [unwired: 17 in]
            }
          }
          n153 = call "BaseProcess.set event status.vi"("i ref in"=w400, "EventStatus"=w397, "error in (no error)"=w399) -> ("i ref out"=w396:refnum<vi>, "error out"=w398:errorcluster)  [unwired: 14 in, 1 out]
          n154 = Unbundle By Name(w398) -> ("code"=w403:i32)
          n155 = case shown="Error" w398 {
            selector: w398 -> [_ w408]
            tunnel: [_ w406] -> w391
            frame No Error {
            }
            frame Error {
              n156 = Unbundle By Name(w408) -> ("source"=w407:string)
              n157 = call-poly "CoreLib.data 2 byte array.vi"("string"=w407) -> ("byteArray out"=w406:T1)  [unwired: 18 in]
            }
          }
          n158 = Bundle By Name(cluster=w402, "Data"=w391, "Error #"=w403) -> (w401:T2)
        }
        frame "CamType" {
          n159 = Unbundle By Name(w429) -> ("Data"=w421:T1)
          n160 = call-poly "CoreLib.byte array 2 data.vi"("byteArray"=w421) -> ("i16"=w422:i16, "error out"=w419:errorcluster)  [unwired: 16 in, 1 out]
          n161 = Not Equal To 0?(x=w422) -> (x != 0?=w420:bool)
          n162 = case shown="No Error" w419 {
            tunnel: [w437 w444] -> w427
            tunnel: w432 -> [w440 w444]
            tunnel: w431 -> [w439 w443]
            tunnel: [w438 w442] -> w426
            tunnel: w424 -> [_ w441]
            tunnel: w420 -> [w436 _]
            frame No Error {
              n163 = call "PH_ImageOperator.PC CamType.vi"("i ref in"=w440, "Nearfield/Farfield"=w436, "error in (no error)"=w439) -> ("i ref out"=w437:refnum<vi>, "error out"=w438:errorcluster)  [unwired: 15 in]
            }
            frame Error {
              n164 = call "CoreLib.set data type mismatch.vi"("error in (no error)"=w443, "error source"=w441) -> ("error out"=w442:errorcluster)  [unwired: 17 in]
            }
          }
          n165 = call "BaseProcess.set event status.vi"("i ref in"=w427, "EventStatus"=w424, "error in (no error)"=w426) -> ("i ref out"=w423:refnum<vi>, "error out"=w425:errorcluster)  [unwired: 14 in, 1 out]
          n166 = Unbundle By Name(w425) -> ("code"=w430:i32)
          n167 = case shown="Error" w425 {
            selector: w425 -> [_ w435]
            tunnel: [_ w433] -> w418
            frame No Error {
            }
            frame Error {
              n168 = Unbundle By Name(w435) -> ("source"=w434:string)
              n169 = call-poly "CoreLib.data 2 byte array.vi"("string"=w434) -> ("byteArray out"=w433:T1)  [unwired: 18 in]
            }
          }
          n170 = Bundle By Name(cluster=w429, "Data"=w418, "Error #"=w430) -> (w428:T2)
        }
        frame "SetCenter" {
          w455 = 2 ("y")
          n171 = call "PH_ImageOperator.get i attribute.vi"("i ref in"=w462, "error in (no error)"=w460) -> ("i ref out"=w461:refnum<vi>, "i attribute"=w459:T5, "error out"=w449:errorcluster)  [unwired: 15 in]
          n172 = Unbundle By Name(w459) -> ("Images.OP"=w445:T9, "GUI Refs.Center"=w447:refnum<vi>)
          n173 = Not A Number/Path/Refnum?(number/path/refnum=w447) -> (NaN/Path/Refnum?=w448:bool)
          n174 = case shown="False" w448 {
            selector: w448 -> [w471 _]
            tunnel: [w474 w475] -> w450
            tunnel: w449 -> [w473 w475]
            tunnel: w447 -> [w472 _]
            frame False {
              n175 = property class="Bool (strict)"(reference=w472, error in=w473, "Value"=w471) -> (error out=w474:errorcluster)  [unwired: 1 out]
            }
            frame True {
            }
          }
          n176 = call "IMAQ GetImageSize"("Image"=w445, "error in (no error)"=w450) -> ("Y Resolution"=w456:i32, "X Resolution"=w457:i32, "error out"=w458:errorcluster)  [unwired: 2 in]
          n177 = Divide(x=w457, y=w455) -> (x/y=w454:dbl)
          n178 = Divide(x=w456, y=w455) -> (x/y=w453:dbl)
          n179 = To Long Integer(number=w454) -> (32bit integer=w451:i32)
          n180 = To Long Integer(number=w453) -> (32bit integer=w452:i32)
          n181 = call "PH_ImageOperator.PC Set Position Expectiation Values.vi"("i ref in"=w461, "expected X"=w451, "expected Y"=w452, "error in (no error)"=w458) -> ("i ref out"=w467:refnum<vi>, "error out"=w466:errorcluster)  [unwired: 14 in]
          n182 = call "BaseProcess.set event status.vi"("i ref in"=w467, "EventStatus"=w464, "error in (no error)"=w466) -> ("i ref out"=w463:refnum<vi>, "error out"=w465:errorcluster)  [unwired: 14 in, 1 out]
          n183 = Unbundle By Name(w465) -> ("code"=w470:i32)
          n184 = case shown="Error" w465 {
            selector: w465 -> [_ w478]
            tunnel: [_ w476] -> w446
            frame No Error {
            }
            frame Error {
              n185 = Unbundle By Name(w478) -> ("source"=w477:string)
              n186 = call-poly "CoreLib.data 2 byte array.vi"("string"=w477) -> ("byteArray out"=w476:T1)  [unwired: 18 in]
            }
          }
          n187 = Bundle By Name(cluster=w469, "Data"=w446, "Error #"=w470) -> (w468:T2)
        }
        frame "SetTraceAnalOn" {
          n188 = Unbundle By Name(w490) -> ("Data"=w482:T1)
          n189 = call-poly "CoreLib.byte array 2 data.vi"("byteArray"=w482) -> ("i16"=w483:i16, "error out"=w480:errorcluster)  [unwired: 16 in, 1 out]
          n190 = Not Equal To 0?(x=w483) -> (x != 0?=w481:bool)
          n191 = case shown="No Error" w480 {
            tunnel: [w499 w505] -> w488
            tunnel: w493 -> [w500 w505]
            tunnel: w492 -> [w501 w504]
            tunnel: [w498 w503] -> w487
            tunnel: w485 -> [_ w502]
            tunnel: w481 -> [w497 _]
            frame No Error {
              n192 = call "PH_ImageOperator.PC set Trace Analysis.vi"("i ref in"=w500, "Trace Analysis on"=w497, "error in (no error)"=w501) -> ("i ref out"=w499:refnum<vi>, "error out"=w498:errorcluster)  [unwired: 15 in]
            }
            frame Error {
              n193 = call "CoreLib.set data type mismatch.vi"("error in (no error)"=w504, "error source"=w502) -> ("error out"=w503:errorcluster)  [unwired: 17 in]
            }
          }
          n194 = call "BaseProcess.set event status.vi"("i ref in"=w488, "EventStatus"=w485, "error in (no error)"=w487) -> ("i ref out"=w484:refnum<vi>, "error out"=w486:errorcluster)  [unwired: 14 in, 1 out]
          n195 = Unbundle By Name(w486) -> ("code"=w491:i32)
          n196 = case shown="Error" w486 {
            selector: w486 -> [_ w496]
            tunnel: [_ w494] -> w479
            frame No Error {
            }
            frame Error {
              n197 = Unbundle By Name(w496) -> ("source"=w495:string)
              n198 = call-poly "CoreLib.data 2 byte array.vi"("string"=w495) -> ("byteArray out"=w494:T1)  [unwired: 18 in]
            }
          }
          n199 = Bundle By Name(cluster=w490, "Data"=w479, "Error #"=w491) -> (w489:T2)
        }
        frame "GaussFitOn" {
          n200 = Unbundle By Name(w517) -> ("Data"=w509:T1)
          n201 = call-poly "CoreLib.byte array 2 data.vi"("byteArray"=w509) -> ("i16"=w510:i16, "error out"=w507:errorcluster)  [unwired: 16 in, 1 out]
          n202 = Not Equal To 0?(x=w510) -> (x != 0?=w508:bool)
          n203 = case shown="No Error" w507 {
            tunnel: [w527 w532] -> w515
            tunnel: w520 -> [w528 w532]
            tunnel: w519 -> [w526 w531]
            tunnel: [w525 w530] -> w514
            tunnel: w512 -> [_ w529]
            tunnel: w508 -> [w524 _]
            frame No Error {
              n204 = call "PH_ImageOperator.PC set Fit.vi"("i ref in"=w528, "Gauss Fit on"=w524, "error in (no error)"=w526) -> ("i ref out"=w527:refnum<vi>, "error out"=w525:errorcluster)  [unwired: 15 in]
            }
            frame Error {
              n205 = call "CoreLib.set data type mismatch.vi"("error in (no error)"=w531, "error source"=w529) -> ("error out"=w530:errorcluster)  [unwired: 17 in]
            }
          }
          n206 = call "BaseProcess.set event status.vi"("i ref in"=w515, "EventStatus"=w512, "error in (no error)"=w514) -> ("i ref out"=w511:refnum<vi>, "error out"=w513:errorcluster)  [unwired: 14 in, 1 out]
          n207 = Unbundle By Name(w513) -> ("code"=w518:i32)
          n208 = case shown="Error" w513 {
            selector: w513 -> [_ w523]
            tunnel: [_ w522] -> w506
            frame No Error {
            }
            frame Error {
              n209 = Unbundle By Name(w523) -> ("source"=w521:string)
              n210 = call-poly "CoreLib.data 2 byte array.vi"("string"=w521) -> ("byteArray out"=w522:T1)  [unwired: 18 in]
            }
          }
          n211 = Bundle By Name(cluster=w517, "Data"=w506, "Error #"=w518) -> (w516:T2)
        }
        frame "NoOffset" {
          n212 = Unbundle By Name(w544) -> ("Data"=w536:T1)
          n213 = call-poly "CoreLib.byte array 2 data.vi"("byteArray"=w536) -> ("i16"=w537:i16, "error out"=w534:errorcluster)  [unwired: 16 in, 1 out]
          n214 = Not Equal To 0?(x=w537) -> (x != 0?=w535:bool)
          n215 = case shown="No Error" w534 {
            tunnel: [w554 w559] -> w542
            tunnel: w547 -> [w555 w559]
            tunnel: w546 -> [w553 w558]
            tunnel: [w552 w557] -> w541
            tunnel: w539 -> [_ w556]
            tunnel: w535 -> [w551 _]
            frame No Error {
              n216 = call "PH_ImageOperator.PC No Offset.vi"("i ref in"=w555, "No Offset"=w551, "error in (no error)"=w553) -> ("i ref out"=w554:refnum<vi>, "error out"=w552:errorcluster)  [unwired: 15 in]
            }
            frame Error {
              n217 = call "CoreLib.set data type mismatch.vi"("error in (no error)"=w558, "error source"=w556) -> ("error out"=w557:errorcluster)  [unwired: 17 in]
            }
          }
          n218 = call "BaseProcess.set event status.vi"("i ref in"=w542, "EventStatus"=w539, "error in (no error)"=w541) -> ("i ref out"=w538:refnum<vi>, "error out"=w540:errorcluster)  [unwired: 14 in, 1 out]
          n219 = Unbundle By Name(w540) -> ("code"=w545:i32)
          n220 = case shown="Error" w540 {
            selector: w540 -> [_ w550]
            tunnel: [_ w548] -> w533
            frame No Error {
            }
            frame Error {
              n221 = Unbundle By Name(w550) -> ("source"=w549:string)
              n222 = call-poly "CoreLib.data 2 byte array.vi"("string"=w549) -> ("byteArray out"=w548:T1)  [unwired: 18 in]
            }
          }
          n223 = Bundle By Name(cluster=w544, "Data"=w533, "Error #"=w545) -> (w543:T2)
        }
        frame "ReadCaliData" {
          n224 = call "PH_ImageOperator.PC Read Cali Data.vi"("i ref in"=w564, "error in (no error)"=w563) -> ("i ref out"=w561:refnum<vi>, "error out"=w562:errorcluster)  [unwired: 16 in]
          n225 = call "BaseProcess.set event status.vi"("i ref in"=w561, "EventStatus"=w566, "error in (no error)"=w562) -> ("i ref out"=w565:refnum<vi>, "error out"=w567:errorcluster)  [unwired: 14 in, 1 out]
          n226 = Unbundle By Name(w567) -> ("code"=w570:i32)
          n227 = case shown="No Error" w567 {
            selector: w567 -> [_ w573]
            tunnel: [_ w571] -> w560
            frame No Error {
            }
            frame Error {
              n228 = Unbundle By Name(w573) -> ("source"=w572:string)
              n229 = call-poly "CoreLib.data 2 byte array.vi"("string"=w572) -> ("byteArray out"=w571:T1)  [unwired: 18 in]
            }
          }
          n230 = Bundle By Name(cluster=w569, "Data"=w560, "Error #"=w570) -> (w568:T2)
        }
        frame "_set_PSDB_Data" {
          n231 = call "CAEObj.unfold trend data.vi"("i ref in"=w577, "raw trend data"=w574) -> ("quality"=w579:i32, "no link"=w582:bool, "data"=w580:i8[], "typeDescriptor"=w581:string, "error out"=w583:errorcluster)  [unwired: 9 in, 4 out]
          n232 = case shown="No Error" w583 {
            tunnel: w578 -> [w603 w613]
            tunnel: [w602 w612] -> w576
            tunnel: [w601 w613] -> w575
            tunnel: w577 -> [w599 w612]
            tunnel: w582 -> [w593 _]
            tunnel: w581 -> [w595 _]
            tunnel: w580 -> [w596 _]
            tunnel: w579 -> [w594 _]
            frame No Error {
              n233 = call "PH_PSDBWriter.get Subsystem DIM Service.vi"("no link"=w593, "typeDescriptor"=w595, "data"=w596, "quality"=w594) -> ("PHELIX Subsystems"=w592:T10)
              n234 = call "PH_PSDBWriter.check PSDB writing condition.vi"("i ref in"=w599, "wanted Subsystem"=w592, "error IO"=w603) -> ("i ref out"=w598:refnum<vi>, "write PSDB?"=w597:bool, "error out"=w600:errorcluster)  [unwired: 14 in]
              n235 = case shown="True" w597 {
                tunnel: w600 -> [w604 w611]
                tunnel: [w605 w608] -> w602
                tunnel: [w604 w606] -> w601
                tunnel: w598 -> [w605 w610]
                frame False {
                }
                frame True {
                  n236 = call "PH_ImageOperator.PC Write PSDB.vi"("i ref in"=w610, "error IO"=w611) -> ("i ref out"=w609:refnum<vi>, "error out"=w607:errorcluster)  [unwired: 16 in]
                  n237 = call "PH_PSDBWriter.evt call write PSDB.vi"("i ref in"=w609, "error in (no error)"=w607) -> ("i ref out"=w608:refnum<vi>, "error out"=w606:errorcluster)  [unwired: 16 in]
                }
              }
            }
            frame Error {
            }
          }
          n238 = call "BaseProcess.set event status.vi"("i ref in"=w576, "EventStatus"=w586, "error in (no error)"=w575) -> ("i ref out"=w587:refnum<vi>, "error out"=w588:errorcluster)  [unwired: 14 in, 1 out]
          n239 = Unbundle By Name(w588) -> ("code"=w591:i32)
          n240 = case shown="No Error" w588 {
            selector: w588 -> [_ w617]
            tunnel: [T1 [] ("byteArray out") w615] -> w585
            frame No Error {
            }
            frame Error {
              n241 = Unbundle By Name(w617) -> ("source"=w616:string)
              n242 = call-poly "CoreLib.data 2 byte array.vi"("string"=w616) -> ("byteArray out"=w615:T1)  [unwired: 18 in]
            }
          }
          n243 = Bundle By Name(cluster=w590, "Data"=w585, "Error #"=w591, "Data Descriptor"="C:N") -> (w589:T2)
        }
      }
    }
    frame Error {
    }
  }
  "answer cluster" <- w7
  "i ref out" <- w5
  "error out" <- w4
